vi "Memory manager V5.vi"   [LabVIEW 2015]
uses:
  <vilib>/Platform/TimedLoop/XDataNode/timing_clust.ctl
  <vilib>/Platform/TimedLoop/XDataNode/nitl_modes.ctl
  <vilib>/Platform/TimedLoop/XDataNode/wakeup.ctl
  <vilib>/rvi/Emulation/niFpgaSctlEmulationGetInTimedLoop.vi
  <vilib>/rvi/Emulation/niFpgaEmulationReportErrorSimple.vi
  <vilib>/rvi/Emulation/niFpgaGetClockAttributes.vi
  <vilib>/rvi/Emulation/niFpgaCriticalErrorInLSC.vi
  LIDAR Slave Globals.vi
  <vilib>/rvi/Emulation/niFpgaEmulationIsFPGAContextNoSignature.vi
  <vilib>/rvi/errors/niFpgaSetErrorForExecOnDevCompSimple.vi
  <vilib>/rvi/eio/common/nirviEmuReportErrorAndStop.vi
  <vilib>/rvi/DataTransferAndStorage/Container/Common/niFpgaContainerGetUniqueNameForEmu.vi
  <vilib>/rvi/FIFO/Fifo_Resource/nirvififoEmulationSetSize.vi
  <vilib>/rvi/FIFO/Fifo_Resource/nirviFifoEmulationQueueMgr.vi
  <instcachedir>/0/nirviFifoEmulationQueueMgr_E5CAEC123FF24DC58D834DCA3CDAA9B5.lvgen/nirviFifoEmulationQueueMgr_E5CAEC123FF24DC58D834DCA3CDAA9B5_001.vi
  <vilib>/Utility/error.llb/Clear Errors.vi
  <vilib>/rvi/FIFO/Fifo_Resource/nirvififoEmulationCreateLock.vi
  <vilib>/rvi/Emulation/niFpgaProcessEmulError.vi
  <vilib>/rvi/FIFO/Fifo_Resource/nirvififoEmulationObtainLock.vi
  <vilib>/rvi/FIFO/Fifo_Resource/nirvififoEmulationReleaseLock.vi
  <vilib>/rvi/occurrence/nirviWaitOnOccurrenceBase.vi
  <vilib>/rvi/errors/nirviReportUnexpectedCaseInternalError.vi
  <vilib>/rvi/errors/nirviReportUnexpectedCaseInternalError (U32).vi
  <vilib>/rvi/Memory/Memory_Emulation/nirvimemoryFastEmulation.vi
  <vilib>/rvi/Memory/Memory_Emulation/nirvimemoryEmulation.vi
  <vilib>/rvi/FIFO/Fifo_Resource/nirvififoEmulationDetermineInputValidOut.vi
  <vilib>/Platform/TimedLoop/XDataNode/XDataNode.xnode
  <vilib>/rvi/DataTransferAndStorage/Container/XNode/niFpgaContainer.xnode
  <vilib>/rvi/FIFO/Fifo_Resource/nirvififoEmulationRead.vi
  <vilib>/rvi/FIFO/Fifo_Resource/nirvififoEmulationWrite.vi
  <vilib>/rvi/FXPMathLib/FxpAdd/XNode/nifxpmath_Add.xnode
  <vilib>/Platform/TimedLoop/XDataNode/XDNodeRunTimeDep.lvlib
  <vilib>/rvi/FXPMathLib/sim/FxpSim.dll
types:
  T1 = typedef "XDNodeRunTimeDep.lvlib/timing_clust.ctl" = cluster{"Expected End [f-1]":u64, "Actual End [f-1]":u64, "Finished Late? [f-1]":bool, "Expected End [i-1]":u64, "Actual End [i-1]":u64, "Finished Late? [i-1]":bool, "Expected Start [i]":u64, "Actual Start [i]":u64, "Expected Start [f]":u64, "Actual Start [f]":u64, "Source Name":string, "Structure Name":string, "Period":i64, "Deadline":i64, "Offset":i64, "Start":i64, "Priority":i32, "Timeout":i32, "Mode":T2, "Wakeup Reason":T3, "Error":errorcluster, "Source Type":string, "Secondary Source Type":string, "Global End Time":u64, "Global Start Time":u64, "Frame Duration":u64, "Iteration Duration":u64, "Assigned CPU":i32, "I/O Scan Engine Mode":u32}
  T2 = typedef "XDNodeRunTimeDep.lvlib/nitl_modes.ctl" = enum32{"No Change", "Process missed periods, maintain original phase", "Discard missed periods, maintain original phase", "Process missed periods, ignore original phase", "Discard missed periods, ignore original phase"}
  T3 = typedef "XDNodeRunTimeDep.lvlib/wakeup.ctl" = enum32{"Normal", "Aborted", "Asynchronous wakeup", "Timing source error", "Timed loop error", "Timeout"}
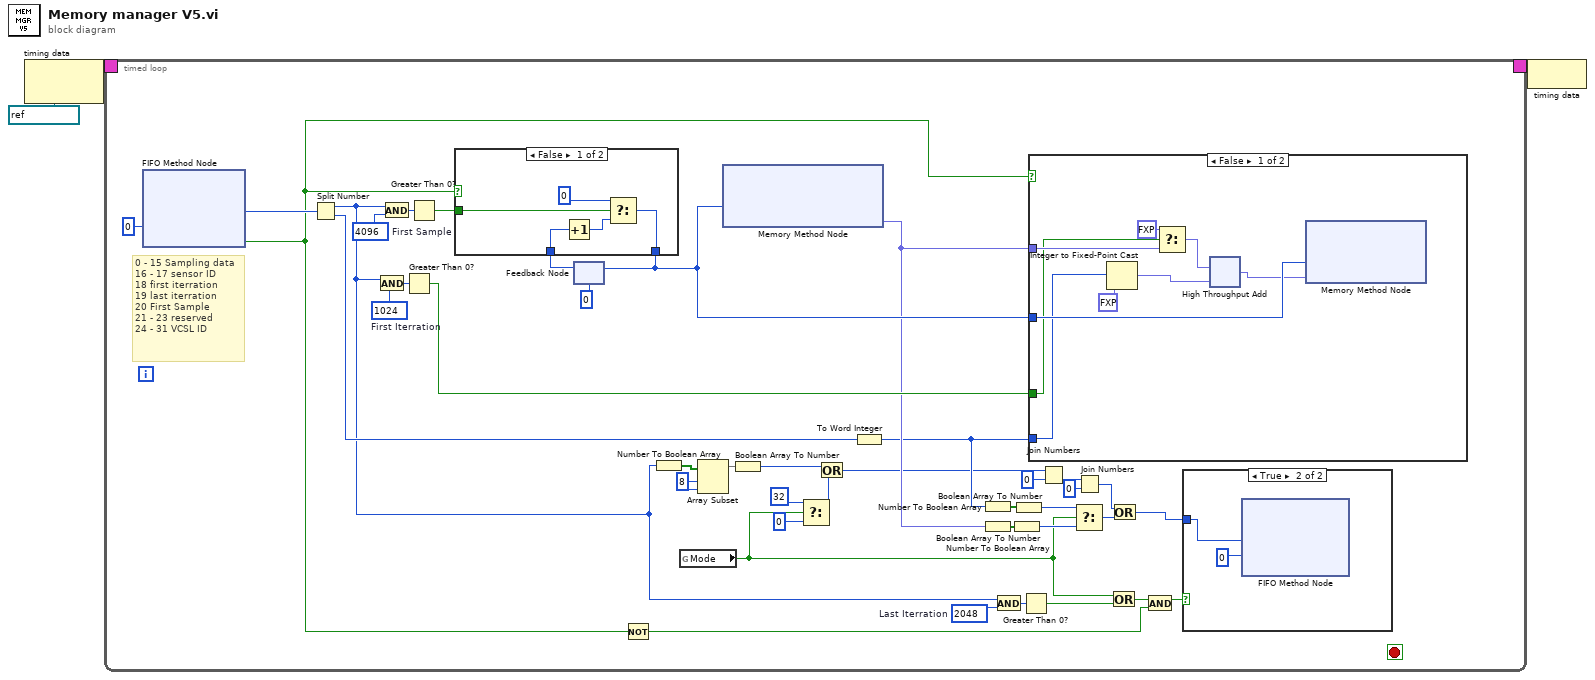
[diagram p0: block diagram]
diagram:
  n1 = node-c288(refnum<k21> "130MHz" ("Source Name")) -> (w3:T1)
  n2 = timed-loop {
    timing: w3 -> [_]
    timing-out: [_] -> w2
    stop <- _ stop-if-true
    w12 = 8 ("index")
    w31 = u16 1024  # First Iterration
    w37 = u16 2048  # Last Iterration
    w40 = u16 4096  # First Sample
    # "0 - 15 Sampling data\n16 - 17 sensor ID\n18 first iterration\n19 last iterration\n20 First Sample\n21 - 23 reserved\n24 - 31 VCSL ID"
    n3 = xnode ("FIFO Method Node")("Timeout"=0) -> ("Element"=w28:u32, "Timed Out?"=w27:bool)  [unwired: 1 in, 1 out]
    n4 = Split Number(x=w28) -> (hi(x)=w13:u16, lo(x)=w39:u16)
    n5 = And(x=w13, y=w31) -> (x .and. y?=w32:u16)
    n6 = And(x=w13, y=w40) -> (x .and. y?=w41:u16)
    n7 = Greater Than 0?(x=w32) -> (x > 0?=w29:bool)
    n8 = Greater Than 0?(x=w41) -> (x > 0?=w30:bool)
    n9 = feedback #1(u32 0 ("Element")) -> (w42:u32)
    n10 = case shown="False" w27 {
      tunnel: [w59 w61] -> w26
      tunnel: w42 -> [w58 w61]
      tunnel: w30 -> [w56 _]
      frame False {
        n11 = Increment(x=w58) -> (x+1=w57:u32)
        n12 = Select(t=u32 0 ("Element"), s=w56, f=w57) -> (s? t:f=w59:u32)
      }
      frame True {
      }
    }
    n13 = feedback-in #1(w26) -> ()
    n14 = Not(x=w27) -> (.not. x?=w33:bool)
    n15 = Number To Boolean Array(number=w13) -> (Boolean array=w11:bool[])
    n16 = global read "LIDAR Slave Globals.vi" "Mode"() -> (w4:bool)
    n17 = Array Subset(array=w11, index=w12, length=w12) -> (w10:bool[])
    n18 = xnode ("Memory Method Node")("Address"=w26) -> ("Data"=w21:fxp<+/-,22,22>)  [unwired: 1 in, 1 out]
    n19 = Boolean Array To Number(Boolean array=w10) -> (number=w9:u8)
    n20 = Select(t=u8 32 ("y"), s=w4, f=u8 0) -> (s? t:f=w6:u8)
    n21 = Or(x=w9, y=w6) -> (x .or. y?=w8:u8)
    n22 = To Word Integer(number=w39) -> (16bit integer=w20:i16)
    n23 = Number To Boolean Array(number=w20) -> (Boolean array=w24:bool[])
    n24 = Number To Boolean Array(number=w21) -> (Boolean array=w22:bool[])
    n25 = And(x=w13, y=w37) -> (x .and. y?=w38:u16)
    n26 = Boolean Array To Number(Boolean array=w22) -> (number=w23:u32)
    n27 = Boolean Array To Number(Boolean array=w24) -> (number=w25:u32)
    n28 = Greater Than 0?(x=w38) -> (x > 0?=w36:bool)
    n29 = case shown="False" w27 {
      tunnel: w21 -> [w54 _]
      tunnel: w20 -> [w47 _]
      tunnel: w26 -> [w52 _]
      tunnel: w29 -> [w48 _]
      frame False {
        n30 = Integer to Fixed-Point Cast(fixed-point type=fxp<+/-,16,16> 0.0, integer=w47) -> (fixed-point=w49:fxp<+/-,16,16>)
        n31 = Select(t=fxp<+/-,22,22> 0.0, s=w48, f=w54) -> (s? t:f=w53:fxp<+/-,22,22>)
        n32 = xnode ("High Throughput Add")("x"=w53, "y"=w49) -> ("x+y"=w51:fxp<+/-,22,22>)
        n33 = xnode ("Memory Method Node")("Address"=w52, "Data"=w51) -> ()  [unwired: 1 in, 1 out]
      }
      frame True {
      }
    }
    n34 = Join Numbers(hi=w8, lo=u8 0) -> ((hi.lo)=w18:u16)
    n35 = Select(t=w25, s=w4, f=w23) -> (s? t:f=w16:u32)
    n36 = Join Numbers(hi=w18, lo=u16 0) -> ((hi.lo)=w15:u32)
    n37 = Or(x=w4, y=w36) -> (x .or. y?=w35:bool)
    n38 = Or(x=w15, y=w16) -> (x .or. y?=w14:u32)
    n39 = And(x=w35, y=w33) -> (x .and. y?=w34:bool)
    n40 = case shown="True" w34 {
      tunnel: w14 -> [_ w45]
      frame False {
      }
      frame True {
        n41 = xnode ("FIFO Method Node")("Element"=w45, "Timeout"=0) -> ()  [unwired: 1 in, 2 out]
      }
    }
  }
  n42 = node-c288(w2) -> ()
